vi "line edge fitting.vi"(8 "error in (no error)":errorcluster, 9 "Paramter guess":dbl[](array[numeric])=[165.0, 0.2, 0.1], 10 "y":dbl[](array[numeric]), 11 "x":dbl[](array[numeric])) -> (0 "error out":errorcluster, 1 "XY Graph":cluster{cdb[]}[](graph), 2 "best nonlinear fit":dbl[](array[numeric]), 3 "best fit parameters":dbl[](array[numeric]))   [LabVIEW 2012, in "LineCCD.lvclass"]
uses:
  LineCCD/LineCCD/LineCCD.lvclass
  <vilib>/gmath/NumericalOptimization/Nonlinear Curve Fit LM.vi
  <vilib>/gmath/NI_Gmath.lvlib
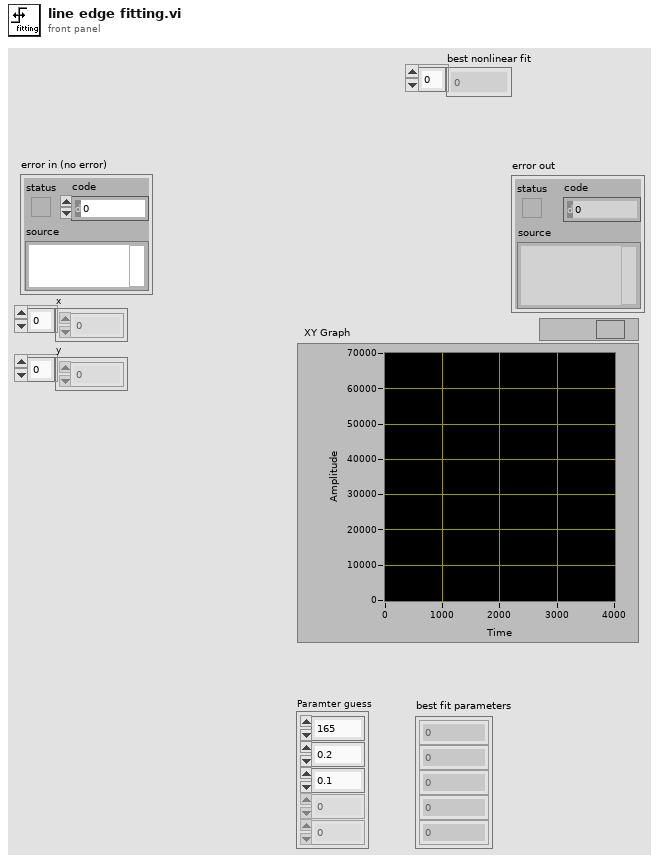
[diagram p1: front panel]
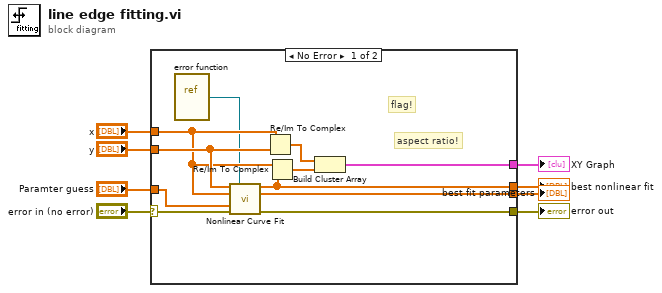
[diagram p0: block diagram]
diagram:
  n1 = case shown="No Error" "error in (no error)" {
    selector: "error in (no error)" -> [w12 w20]
    tunnel: [w17 _] -> w3
    tunnel: "y" -> [w16 _]
    tunnel: "x" -> [w15 _]
    tunnel: "Paramter guess" -> [w14 _]
    tunnel: [w9 w20] -> w4
    tunnel: [w13 _] -> w6
    tunnel: [w10 _] -> w1
    frame No Error {
      # "aspect ratio!"
      # "flag!"
      n2 = vi-ref "error function.vi"() -> (w11:refnum<vi>)
      n3 = call-poly <vilib>:"Nonlinear Curve Fit.vi"("Y"=w16, "f(x,a)"=w11, "X"=w15, "initial parameters"=w14, "error in (no error)"=w12) -> ("best nonlinear fit"=w10:dbl[], "best fit parameters"=w13:dbl[], "error out"=w9:errorcluster)  [unwired: 5 in, 3 out]
      n4 = Re/Im To Complex(1:w16, 2:w15) -> (0:w19:cdb[])
      n5 = Re/Im To Complex(1:w10, 2:w15) -> (0:w18:cdb[])
      n6 = Build Cluster Array(w19, w18) -> (w17:cluster{cdb[]}[])
    }
    frame Error {
    }
  }
  "XY Graph" <- w3
  "error out" <- w4
  "best fit parameters" <- w6
  "best nonlinear fit" <- w1
